vi "ODE-Plot-name-checker.vi"(1 "In Plot Name":string[](array[string])) -> (0 "Out Plot Name":string[](array[string]))   [LabVIEW 2014]
doc: "This VI checks the plot names of VI to avoid repeting legends."
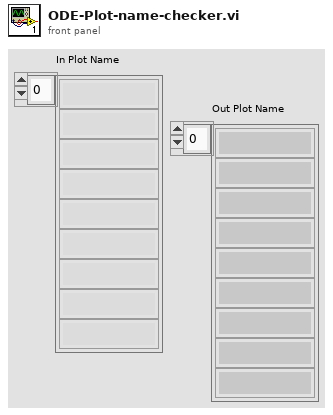
[diagram p1: front panel]
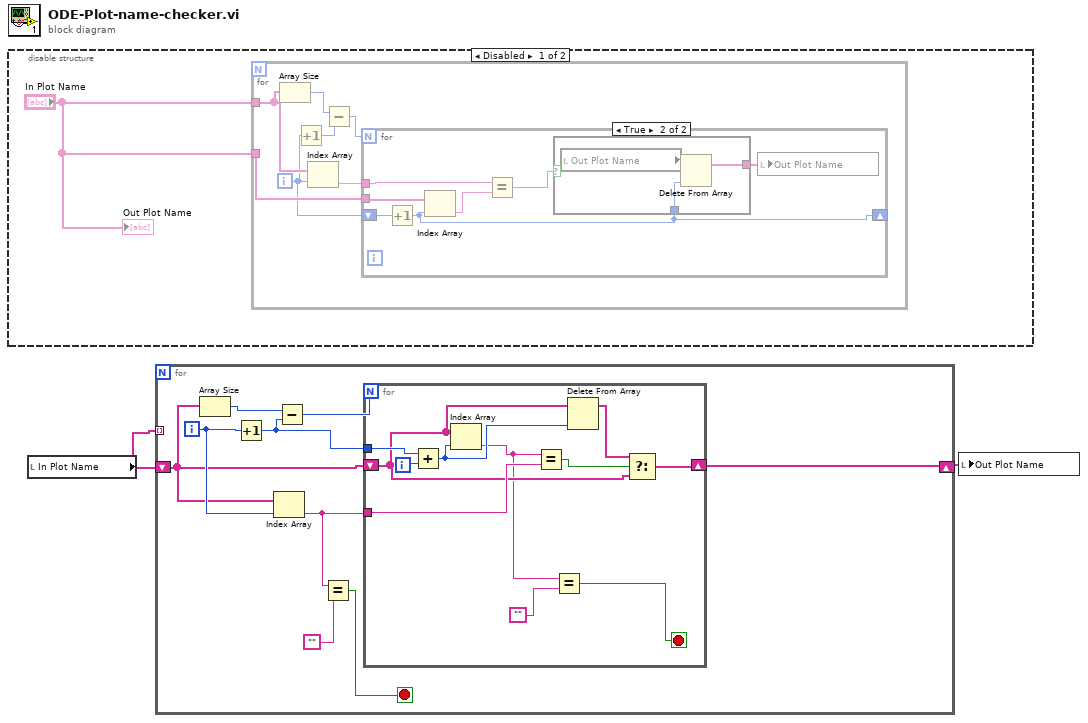
[diagram p0: block diagram]
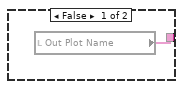
[diagram p2: hidden frame]
diagram:
  n1 = disable-structure shown="Disabled" {
    frame Disabled {
      n2 = for {
        tunnel: "In Plot Name" -> [w10]
        tunnel: "In Plot Name" -> [w9]
        i -> [w7]
        n3 = Array Size(array=w9) -> (size(s)=w5:i32)
        n4 = Increment(x=w7) -> (x+1=w6:i32)
        n5 = Index Array(array=w9, index=w7) -> (element=w8:string)
        n6 = Subtract(x=w5, y=w6) -> (x-y=w4:i32)
        n7 = for {
          N: w4 -> [_]
          tunnel: w10 -> [w17]
          tunnel: w8 -> [w15]
          shift-right: [w11] -> _
          shift-left: w7 -> [w12]
          n8 = Increment(x=w12) -> (x+1=w11:i32)
          n9 = Index Array(array=w17, index=w11) -> (element=w16:string)
          n10 = Equal?(x=w15, y=w16) -> (x = y?=w13:bool)
          n11 = case shown="True" w13 {
            tunnel: [w18 w20] -> w14
            tunnel: w11 -> [_ w19]
            frame False {
              n12 = local read "Out Plot Name"() -> (w18:string[])
            }
            frame True {
              n13 = local read "Out Plot Name"() -> (w21:string[])
              n14 = Delete From Array(array=w21, index=w19) -> (array with subset deleted=w20:string[])  [unwired: 1 in, 1 out]
            }
          }
          n15 = local write "Out Plot Name"(w14) -> ()
        }
      }
      "Out Plot Name" <- "In Plot Name"
    }
    frame Enabled {
    }
  }
  n16 = local read "In Plot Name"() -> (w2:string[])
  n17 = for {
    tunnel: w2 -> [_] mode=indexing
    shift-right: [w23] -> w1
    shift-left: w2 -> [w22]
    i -> [w27]
    stop <- w25 stop-if-true
    n18 = Array Size(array=w22) -> (size(s)=w30:i32)
    n19 = Increment(x=w27) -> (x+1=w28:i32)
    n20 = Index Array(array=w22, index=w27) -> (element=w24:string)
    n21 = Subtract(x=w30, y=w28) -> (x-y=w29:i32)
    n22 = Equal?(x=w24, y="") -> (x = y?=w25:bool)
    n23 = for {
      N: w29 -> [_]
      tunnel: w28 -> [w41]
      tunnel: w24 -> [w39]
      shift-right: [w35] -> w23
      shift-left: w22 -> [w34]
      i -> [w40]
      stop <- w31 stop-if-true
      n24 = Add(x=w41, y=w40) -> (x+y=w37:i32)
      n25 = Index Array(array=w34, index=w37) -> (element=w32:string)
      n26 = Equal?(x=w32, y=w39) -> (x = y?=w38:bool)
      n27 = Equal?(x=w32, y="") -> (x = y?=w31:bool)
      n28 = Delete From Array(array=w34, index=w37) -> (array with subset deleted=w36:string[])  [unwired: 1 in, 1 out]
      n29 = Select(t=w36, s=w38, f=w34) -> (s? t:f=w35:string[])
    }
  }
  n30 = local write "Out Plot Name"(w1) -> ()
